vi "get_archivisation_info_from_DB.vi"(0 "station_number":u16, 1 "name_table":string, 2 "variable_start_index":i32, 4 "station":T1, 5 "error_in":errorcluster, 6 "SQL_connection_reference":T2, 7 "results_from_PLC":u8[](array[numeric])) -> (14 "archivisation_info":string[][](array[string]), 19 "error_out":errorcluster)   [LabVIEW 2020]
uses:
  <vilib>/addons/database/Connection.llb/Conn ObjectReference.ctl
  station.ctl
  _misc/byte_array_parser/to_string.vi
  <vilib>/addons/database/NI_Database_API.lvlib
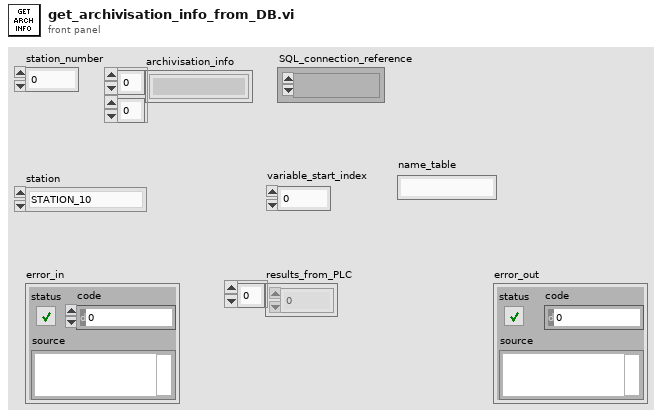
[diagram p1: front panel]
types:
  T1 = typedef "station.ctl" = enum16{"STATION_10", "STATION_20", "STATION_30", "STATION_40", "STATION_50", "STATION_60", "STATION_70", "STATION_80", "STATION_90", "STATION_100", "STATION_110", "STATION_120", "STATION_165", "MAIN"}
  T2 = typedef "NI_Database_API.lvlib/Conn ObjectReference.ctl" = refnum<k1>
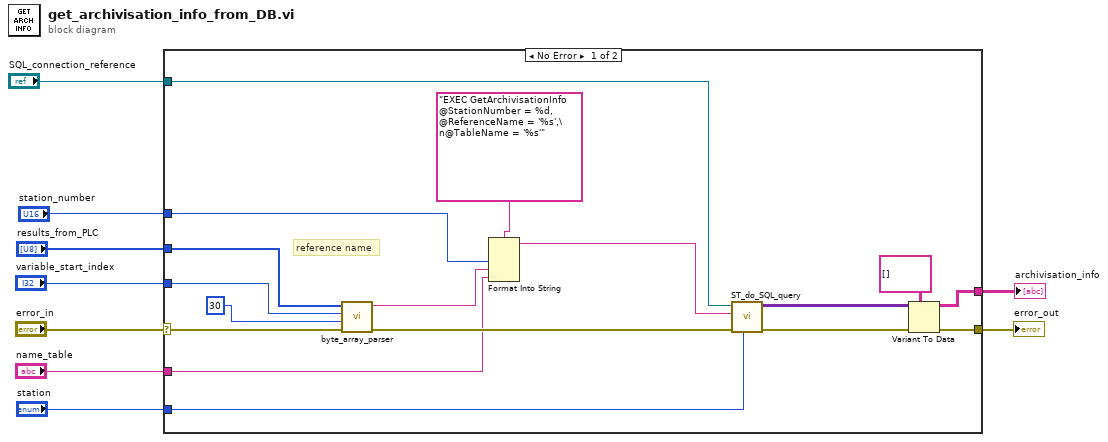
[diagram p0: block diagram]
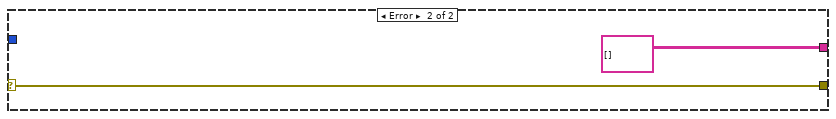
[diagram p2: hidden frame]
diagram:
  n1 = case shown="No Error" "error_in" {
    selector: "error_in" -> [w22 w28]
    tunnel: [w26 string[][] []] -> w9
    tunnel: "SQL_connection_reference" -> [w24 _]
    tunnel: [w15 w28] -> w7
    tunnel: "results_from_PLC" -> [w23 _]
    tunnel: "station_number" -> [w21 _]
    tunnel: "station" -> [w17 _]
    tunnel: "variable_start_index" -> [w13 _]
    tunnel: "name_table" -> [w10 _]
    frame No Error {
      # "reference name"
      n2 = call-poly "byte_array_parser.vi"("error_in"=w22, "string_length"=30, "variable_start_index"=w13, "byte_array"=w23) -> ("error_out"=w16:errorcluster, "string"=w20:string)  [unwired: 6 in]
      n3 = Format Into String(format string="EXEC GetArchivisationInfo @StationNumber = %d, @ReferenceName = '%s',\n@TableName = '%s'", w21, w20, w10) -> (resulting string=w19:string)  [unwired: 2 in, 1 out]
      n4 = call "ST_do_SQL_query.vi"("station"=w17, "error_in"=w16, "SQL_query"=w19, "SQL_connection_reference"=w24) -> ("error_out"=w14:errorcluster, "recordset_out"=w18:variant[][])  [unwired: 6 in]
      n5 = Variant To Data(error in=w14, type=string[][] [], Variant=w18) -> (data=w26:string[][], error out=w15:errorcluster)
    }
    frame Error {
    }
  }
  "archivisation_info" <- w9
  "error_out" <- w7
